vi "SetSMOState.vi"(8 "error in (no error)":errorcluster, 10 "SMO State":T1, 11 "SMO in":refnum<class "SMO.lvclass">) -> (0 "error out":errorcluster, 3 "SMO out":refnum<class "SMO.lvclass">)   [LabVIEW 2019, in "SMO.lvclass"]
doc: "JKI State Machine Objects (SMO) 1.3.0.56\nJKI - JKI\nCopyright (c) 2017, JKI"
uses:
  SMO.lvclass
  Typedefs/SMOState --Enum.ctl
  SMO.lvclass/SMO.ctl
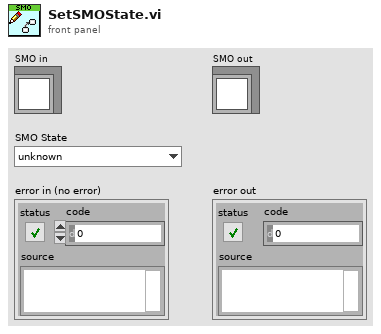
[diagram p1: front panel]
types:
  T1 = typedef "SMO.lvclass/SMOState --Enum.ctl" = enum16{"unknown", "Created", "Started", "Stopped"}
  T2 = typedef "SMO.lvclass/PrivateData--Ref.ctl" = refnum<data-value>
  T3 = typedef "SMO.lvclass/PrivateData--Cluster.ctl" = cluster{"Parent Call":T4, "Registered Processes":T5[], "Sync Notifier":refnum<notifier>, "Process Error Notifier":refnum<notifier>, "Protected Events":T6, "Public Events":T7, "SMO State":T1, "[Dependencies]":T8[], "[Attributes]":refnum<class "Attribute.lvclass">[], "Launcher Close":refnum<notifier>, "Caller Watchdog":refnum<queue>, "Accessibility":T9, "NbStaticDependencies":u32}
  T4 = typedef "SMO.lvclass/Parent Call--Enum.ctl" = enum16{"Allows parent to run", "Does not request parent to run"}
  T5 = typedef "SMO.lvclass/RegisteredProcessData--Cluster.ctl" = cluster{"Name":string, "Static VI Ref":refnum<vi>, "Running":bool, "NotifierRef":u32}
  T6 = typedef "SMO.lvclass/Protected Events.ctl" = cluster{"StopProcesses":refnum<user-event>, "AbortProcesses":refnum<user-event>, "Config Changed":refnum<user-event>, "Dependency":refnum<user-event>}
  T7 = typedef "SMO.lvclass/Public Events.ctl" = cluster{"Error":refnum<user-event>, "State":refnum<user-event>, "Reserve State":refnum<user-event>}
  T8 = typedef "SMO.lvclass/SMO Dependency--Cluster.ctl" = cluster{"Dependency":refnum<class "SMO.lvclass">, "Level":string}
  T9 = typedef "SMO.lvclass/Accessibility--Cluster.ctl" = cluster{"Lock Key":string, "Reserve State":T10}
  T10 = typedef "SMO.lvclass/Reserve State--Enum.ctl" = enum16{"Unreserved", "Reserved", "Self-locked"}
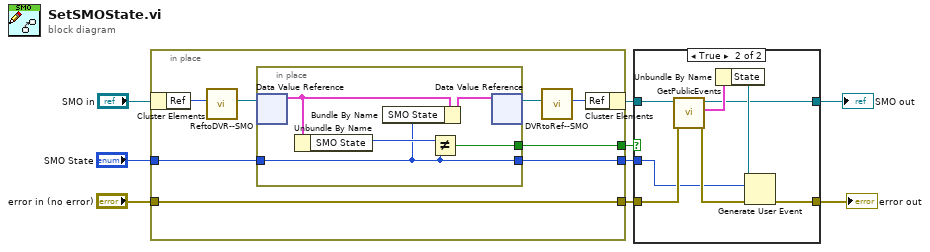
[diagram p0: block diagram]
diagram:
  n1 = in-place {
    in-place-border: "error in (no error)" -> [w17]
    in-place-border: [w17] -> w4
    in-place-border: "SMO State" -> [w12]
    in-place-border: [w11] -> w2
    in-place-border: [w10] -> w1
    n2 = in-place-cluster #1("SMO in") -> ("Ref"=w14:u32)
    n3 = call "ReftoDVR--SMO.vi"("Ref"=w14) -> ("Ref"=w13:T2)  [unwired: 10 in]
    n4 = in-place {
      in-place-border: w12 -> [w19]
      in-place-border: [w19] -> w11
      in-place-border: [w18] -> w10
      n5 = in-place-dvr #2(w13) -> (w22:T3)  [unwired: 1 out]
      n6 = Unbundle By Name(w22) -> ("SMO State"=w20:T1)
      n7 = Bundle By Name(cluster=w22, "SMO State"=w19) -> (w21:T3)
      n8 = Not Equal?(x=w20, y=w19) -> (x != y?=w18:bool)
      n9 = in-place-dvr #2(w21) -> (w15:T2)  [unwired: 1 out]
    }
    n10 = call "DVRtoRef--SMO.vi"("Ref"=w15) -> ("Ref"=w16:u32)  [unwired: 10 in]
    n11 = in-place-cluster #1("Ref"=w16) -> (w6:refnum<class "SMO.lvclass">)
  }
  n12 = case shown="True" w1 {
    tunnel: [w23 w32] -> w9
    tunnel: [w24 w29] -> w8
    tunnel: w6 -> [w24 w27]
    tunnel: w4 -> [w23 w26]
    tunnel: w2 -> [_ w25]
    frame False {
    }
    frame True {
      n13 = call "GetPublicEvents.vi"("error in (no error)"=w26, "SMO"=w27) -> ("error out"=w28:errorcluster, "Public Events"=w30:T7, "SMO out"=w29:refnum<class "SMO.lvclass">)  [unwired: 7 in]
      n14 = Unbundle By Name(w30) -> ("State"=w31:refnum<user-event>)
      n15 = Generate User Event(user event=w31, event data cluster=w25, error in=w28) -> (error out=w32:errorcluster)  [unwired: 1 in, 1 out]
    }
  }
  "error out" <- w9
  "SMO out" <- w8
